vi "hold state logic.vi"(0 "system status in":T2={"system state"=enum."Empty & Closed", "fuel level"=0.0, "LOX level"=0.0, "system warnings"={"oxidizer overpress"=FALSE, "oxidizer leak"=FALSE, "fuel overpress"=FALSE, "fuel leak"=FALSE}, "valves"={"fuel load"=FALSE, "fuel return"=FALSE, "fuel comb"=FALSE, "fuel dump"=FALSE, "LOX load"=FALSE, "LOX return"=FALSE, "LOX comb"=FALSE, "LOX dump"=FALSE}, "ignition"=FALSE}, 7 "rocket controls":T1, 12 "LOX over":bool, 13 "LOX leak":bool, 14 "fuel over":bool, 15 "fuel leak":bool) -> (2 "stop hold loop":bool, 4 "system status out":T2={"system state"=enum."Empty & Closed", "fuel level"=0.0, "LOX level"=0.0, "system warnings"={"oxidizer overpress"=FALSE, "oxidizer leak"=FALSE, "fuel overpress"=FALSE, "fuel leak"=FALSE}, "valves"={"fuel load"=FALSE, "fuel return"=FALSE, "fuel comb"=FALSE, "fuel dump"=FALSE, "LOX load"=FALSE, "LOX return"=FALSE, "LOX comb"=FALSE, "LOX dump"=FALSE}, "ignition"=FALSE}, 8 "rocket controls out":T1)   [LabVIEW 2017]
doc: "This subVI handles the exit logic for the rocket engine simulation Hold state.\nAbort has the highest priroity, then returning lox, returning fuel, shutdown, launch, loading fuel, and loading lox.\n\nPaul K Dixon\nP350\nCSUSB"
uses:
  typedefs/user controls.ctl
  typedefs/sysyem status.ctl
  typedefs/system state.ctl
  typedefs/rocket system warnings.ctl
panel:
  # "Standard\nProcedures"
  # "Alternate\nProcedures"
  # "Standard\nProcedures"
  # "Alternate\nProcedures"
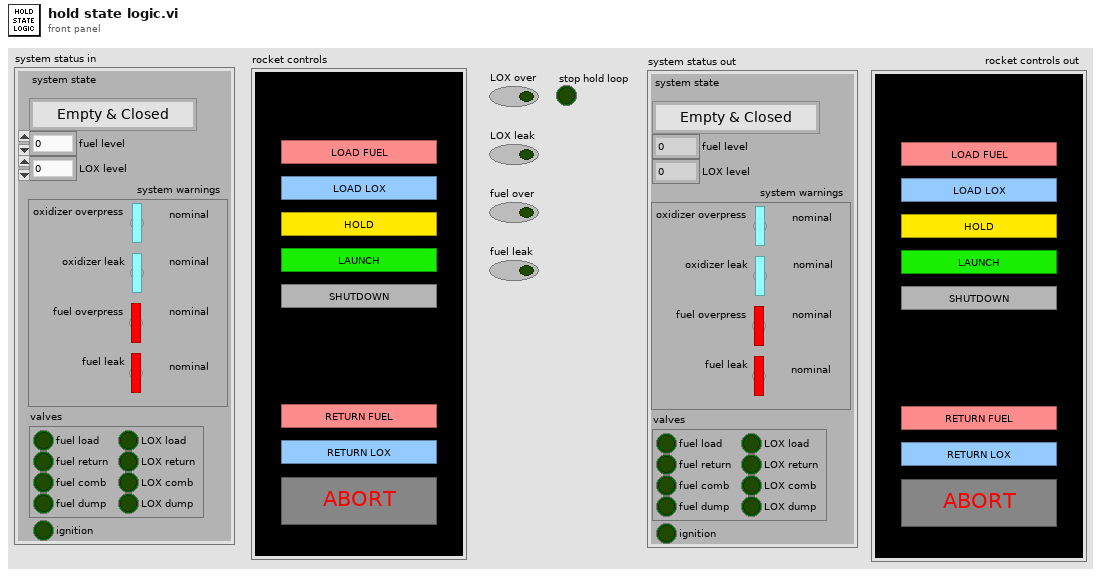
[diagram p1: front panel]
types:
  T1 = typedef "user controls.ctl" = cluster{"load fuel":bool, "load lox":bool, "hold":bool, "launch":bool, "shutdown":bool, "return fuel":bool, "return lox":bool, "abort":bool}
  T2 = typedef "sysyem status.ctl" = cluster{"system state":T3, "fuel level":dbl, "LOX level":dbl, "system warnings":T4, "valves":cluster{"fuel load":bool, "fuel return":bool, "fuel comb":bool, "fuel dump":bool, "LOX load":bool, "LOX return":bool, "LOX comb":bool, "LOX dump":bool}, "ignition":bool}
  T3 = typedef "system state.ctl" = enum16{"Hold", "Empty & Closed", "Launch", "Return Fuel", "Return LOX", "Loading Lox", "Loading Fuel", "Shutdown", "Abort"}
  T4 = typedef "rocket system warnings.ctl" = cluster{"oxidizer overpress":bool, "oxidizer leak":bool, "fuel overpress":bool, "fuel leak":bool}
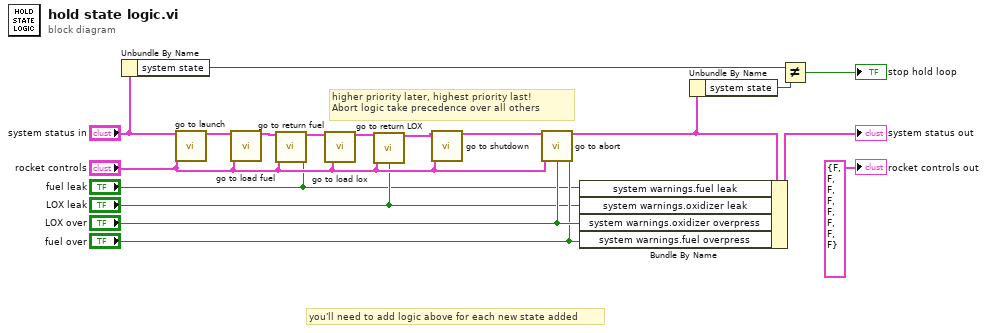
[diagram p0: block diagram]
diagram:
  # "you'll need to add logic above for each new state added"
  # "higher priority later, highest priority last!\nAbort logic take precedence over all others"
  n1 = Unbundle By Name("system status in") -> ("system state"=w16:T3)
  n2 = call "go to launch.vi"("system status in"="system status in", "rocket controls"="rocket controls") -> ("system status out"=w8:T2)  [unwired: 13 in]
  n3 = call "go to load fuel.vi"("system status in"=w8, "rocket controls"="rocket controls") -> ("system status out"=w7:T2)  [unwired: 13 in]
  n4 = call "go to return fuel.vi"("system status in"=w7, "rocket controls"="rocket controls", "fuel leak"="fuel leak") -> ("system status out"=w6:T2)  [unwired: 12 in]
  n5 = call "go to load lox.vi"("system status in"=w6, "rocket controls"="rocket controls") -> ("system status out"=w5:T2)  [unwired: 13 in]
  n6 = call "go to return LOX.vi"("system status in"=w5, "rocket controls"="rocket controls", "LOX leak"="LOX leak") -> ("system status out"=w3:T2)  [unwired: 12 in]
  n7 = call "go to shutdown.vi"("system status in"=w3, "rocket controls"="rocket controls") -> ("system status out"=w10:T2)  [unwired: 13 in]
  n8 = call "go to abort.vi"("system status in"=w10, "rocket controls"="rocket controls", "LOX over"="LOX over", "fuel over"="fuel over") -> ("system status out"=w18:T2)  [unwired: 11 in]
  n9 = Bundle By Name(cluster=w18, "system warnings.fuel leak"="fuel leak", "system warnings.oxidizer leak"="LOX leak", "system warnings.oxidizer overpress"="LOX over", "system warnings.fuel overpress"="fuel over") -> (→"system status out":T2)
  n10 = Unbundle By Name(w18) -> ("system state"=w15:T3)
  n11 = Not Equal?(x=w16, y=w15) -> (x != y?=→"stop hold loop":bool)
  "rocket controls out" <- T1 {"load fuel"=FALSE, "load lox"=FALSE, "hold"=FALSE, "launch"=FALSE, "shutdown"=FALSE, "return fuel"=FALSE, "return lox"=FALSE, "abort"=FALSE} ("rocket controls out")
